vi "ArdnoFeed.vi"(0 "LINX Resource":T2={"IO"=enum."Remote", "Interface"=enum."Serial", "LINX Device Config"={"Interface"=enum."Serial", "COM Port"="COM13", "TCP Configuration"={"IP Address"="", "Port"=0}, "Device Family"=1, "Device ID"=1, "Device Name"="myRIO-1900", "TCP Ref"=refnum, "Channels"={"DI"=[0, 1, 2, 3, 4, 5, 6, 7, 8, 9, 10, 11, 12, 13, 14, 15, 16, 17, 18, 19, 20, 21, 22, 23, 24, 25, 26, 27, 28, 29, 30, 31, 32, 33, 34, 35, 36, 37, 38, 39, 40, 41, 42, 43, 44, 45, 46], "DO"=[0, 1, 2, 3, 4, 5, 6, 7, 8, 9, 10, 11, 12, 13, 14, 15, 16, 17, 18, 19, 20, 21, 22, 23, 24, 25, 26, 27, 28, 29, 30, 31, 32, 33, 34, 35, 36, 37, 38, 39, 40, 41, 42, 43, 44, 45, 46], "AI"=[0, 1, 2, 3, 4, 5, 6, 7, 8, 9, 10, 11], "AO"=[], "PWM"=[3, 5, 6, 9, 10], "QE"=[], "UART"=[0, 1], "I2C 2"=[0], "SPI"=[0], "CAN"=[], "Servo"=[], "AI Ref (V)"=0.0, "AI Resolution (Bits)"=0, "AO Ref (V)"=0.0, "AO Resolution (Bits)"=0}}}, 1 "chip selector":u16(ring) items=["8-Ring", "OneRing", "valveGR"], 5 "Reagent":u32, 7 "Ring":u16, 9 "Feed Cycles":i32, 11 "error in (no error)":errorcluster, 12 "All Rings":bool) -> (4 "LINX Resource out":T2, 6 "Elapsed [ms]":u32, 14 "ValveStates":bool[](array[boolean]), 15 "error out":errorcluster)   [LabVIEW 2018, in "Arduino.lvlib"]
uses:
  Arduino.lvlib
  <vilib>/MakerHub/LINX/Private/Type Defs/LINX Ref.ctl
  <vilib>/MakerHub/LINX/Private/Type Defs/Platform.ctl
  <vilib>/MakerHub/LINX/Private/Type Defs/Interface.ctl
  <vilib>/MakerHub/LINX/Private/Device/Type Defs/LINX Device Config.ctl
  <vilib>/MakerHub/LINX/Private/Device/Type Defs/TCP Config.ctl
  <vilib>/MakerHub/LINX/Private/Device/Type Defs/Channels.ctl
  <vilib>/MakerHub/LINX/Public/Peripherals/Digital/Digital Write N Chans.vi
  <vilib>/MakerHub/LINX/Private/Local IO/LinxDigitalWrite.vi
  <vilib>/MakerHub/LINX/Public/Utilities/Check Channel.vi
  <vilib>/MakerHub/LINX/Private/Utilties/Generate Error.vi
  <vilib>/MakerHub/LINX/LMH-LINX.lvlib
  <vilib>/MakerHub/LINX/Private/Device/Device.lvlib
panel:
  in  "ValveManualCluster":T1
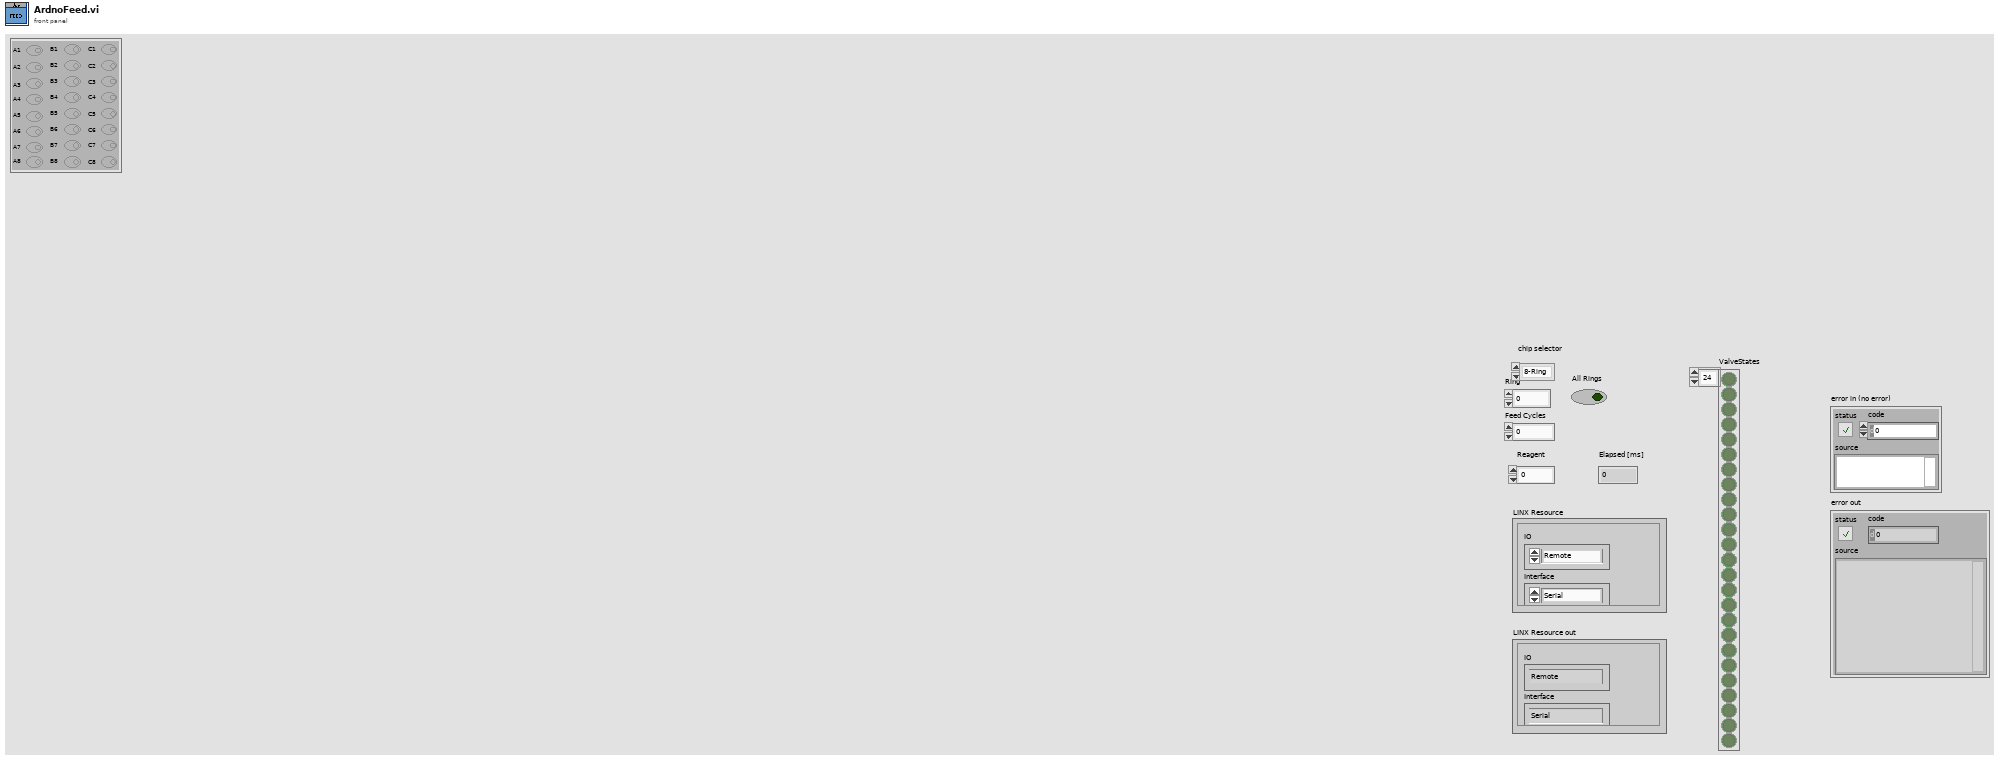
[diagram p1: front panel]
types:
  T1 = cluster{"C8":bool, "C7":bool, "C6":bool, "C5":bool, "C4":bool, "C3":bool, "C2":bool, "C1":bool, "B8":bool, "B7":bool, "B6":bool, "B5":bool, "B4":bool, "B3":bool, "B2":bool, "B1":bool, "A8":bool, "A7":bool, "A6":bool, "A5":bool, "A4":bool, "A3":bool, "A2":bool, "A1":bool}
  T2 = typedef "LMH-LINX.lvlib/LINX Ref.ctl" = cluster{"IO":T3, "Interface":T4, "LINX Device Config":T5}
  T3 = typedef "LMH-LINX.lvlib/Platform.ctl" = enum16{"Remote", "Local"}
  T4 = typedef "LMH-LINX.lvlib/Interface.ctl" = enum16{"Serial", "TCP"}
  T5 = typedef "LMH-LINX.lvlib/Device.lvlib/LINX Device Config.ctl" = cluster{"Interface":T4, "COM Port":refnum<visa-resource-name>, "TCP Configuration":T6, "Device Family":u8, "Device ID":u8, "Device Name":string, "TCP Ref":refnum<k5>, "Channels":T7}
  T6 = typedef "LMH-LINX.lvlib/Device.lvlib/TCP Config.ctl" = cluster{"IP Address":string, "Port":u16}
  T7 = typedef "LMH-LINX.lvlib/Channels.ctl" = cluster{"DI":u8[], "DO":u8[], "AI":u8[], "AO":u8[], "PWM":u8[], "QE":u8[], "UART":u8[], "I2C 2":u8[], "SPI":u8[], "CAN":u8[], "Servo":u8[], "AI Ref (V)":dbl, "AI Resolution (Bits)":u8, "AO Ref (V)":dbl, "AO Resolution (Bits)":u8}
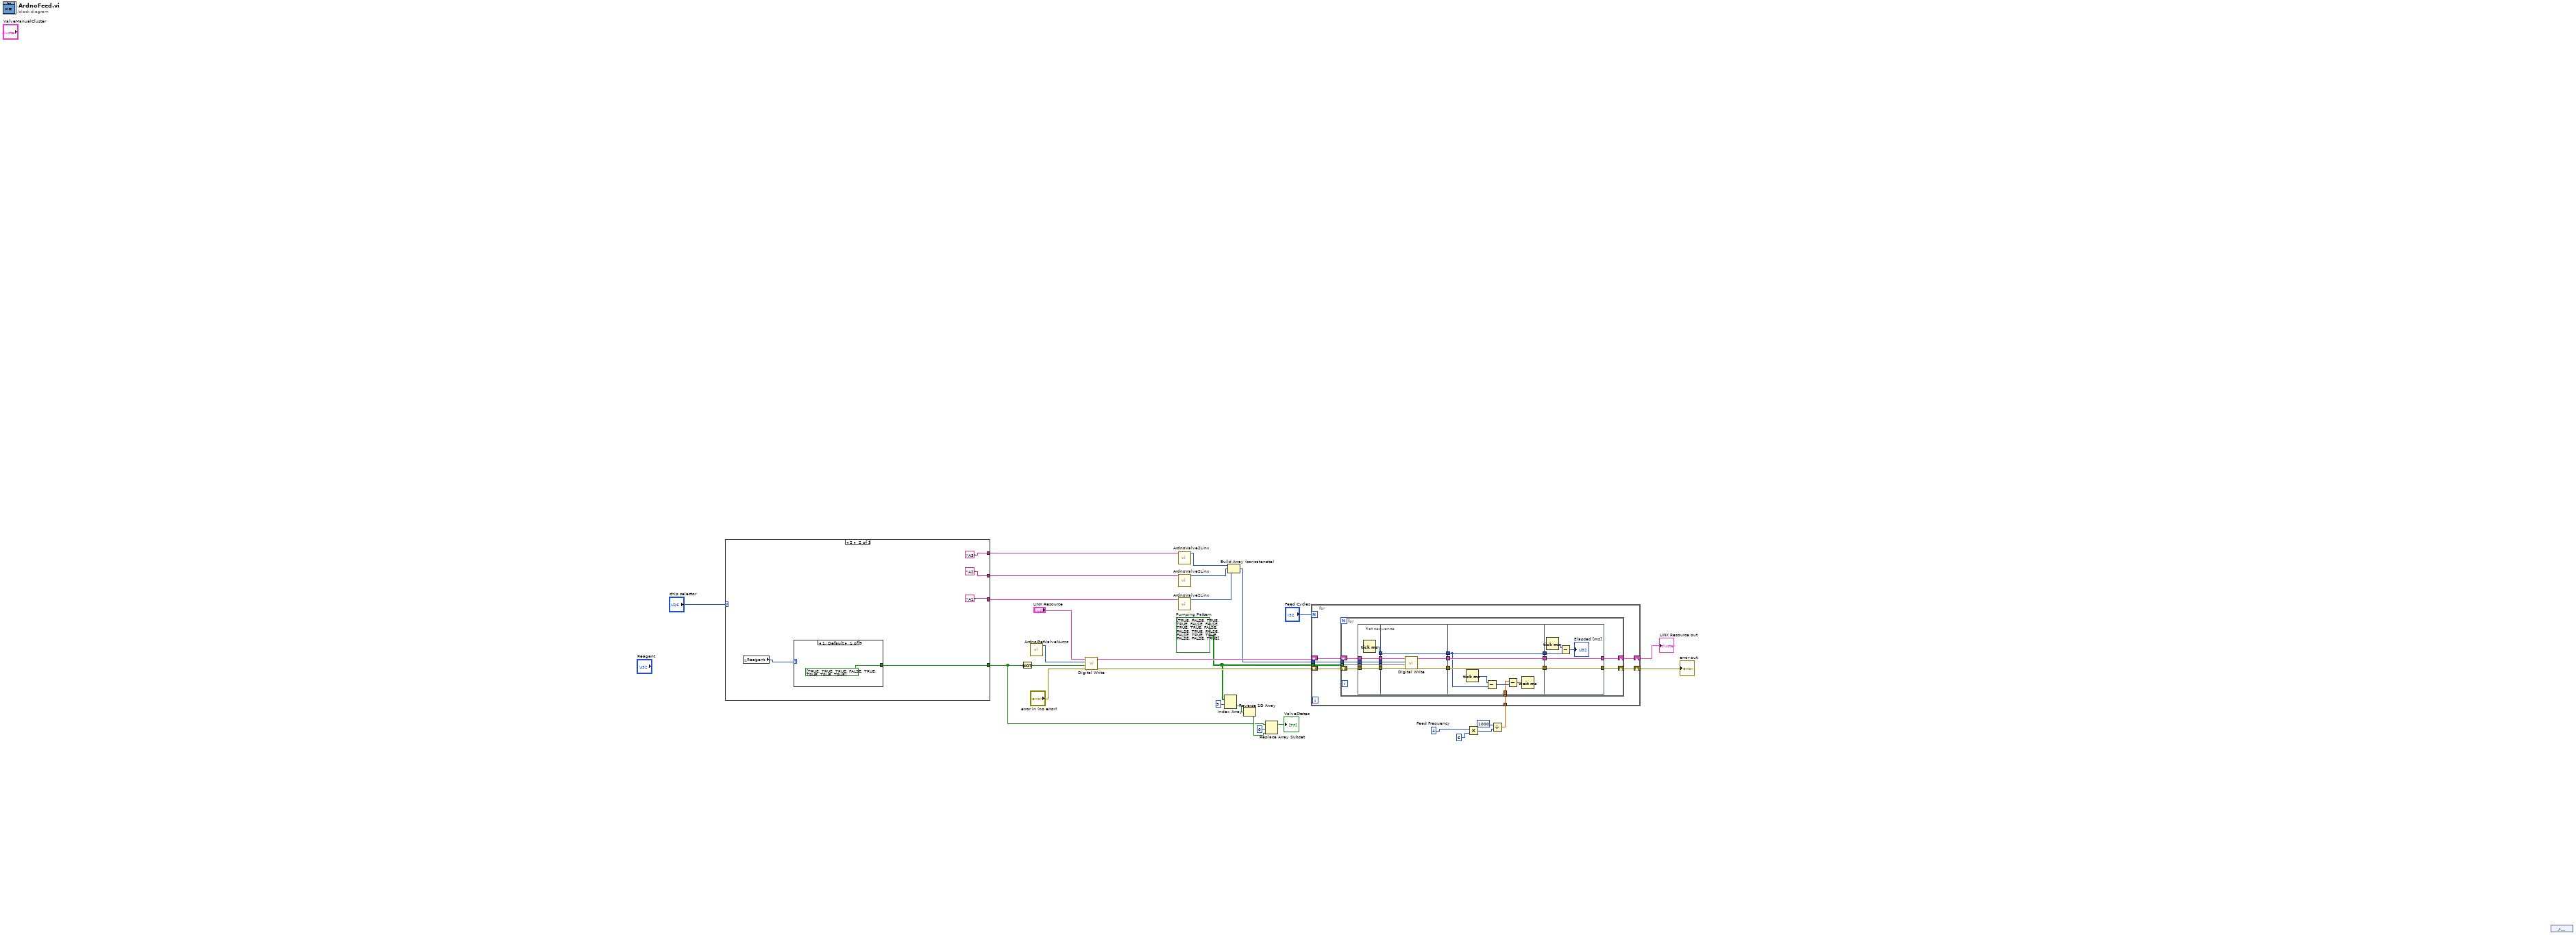
[diagram p0: block diagram]
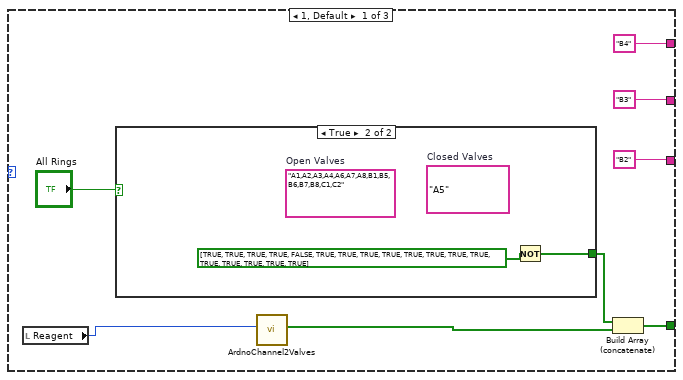
[diagram p2: hidden frame]
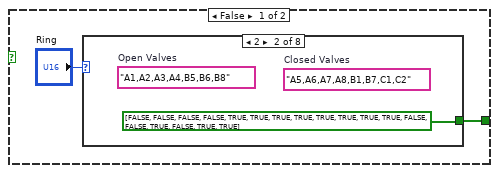
[diagram p3: hidden frame]
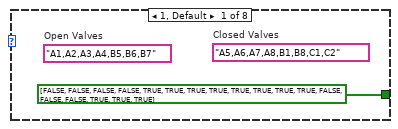
[diagram p4: hidden frame]
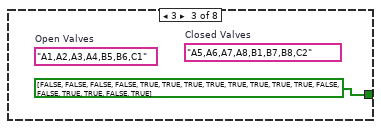
[diagram p5: hidden frame]
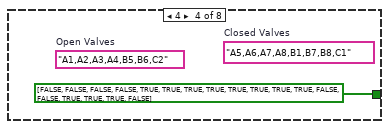
[diagram p6: hidden frame]
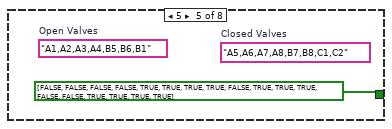
[diagram p7: hidden frame]
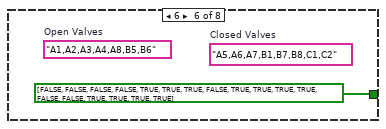
[diagram p8: hidden frame]
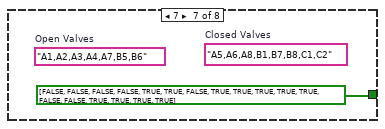
[diagram p9: hidden frame]
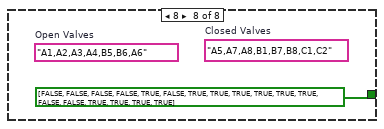
[diagram p10: hidden frame]
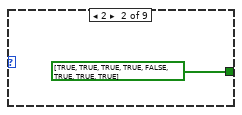
[diagram p11: hidden frame]
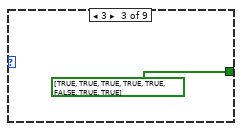
[diagram p12: hidden frame]
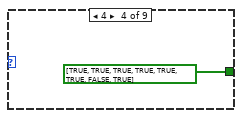
[diagram p13: hidden frame]
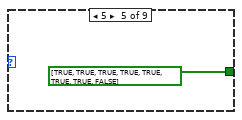
[diagram p14: hidden frame]
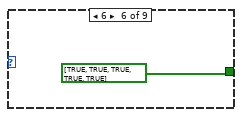
[diagram p15: hidden frame]
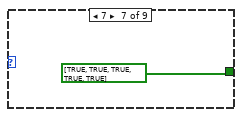
[diagram p16: hidden frame]
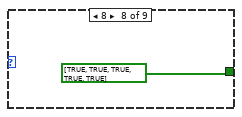
[diagram p17: hidden frame]
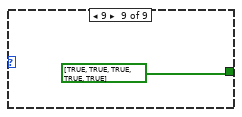
[diagram p18: hidden frame]
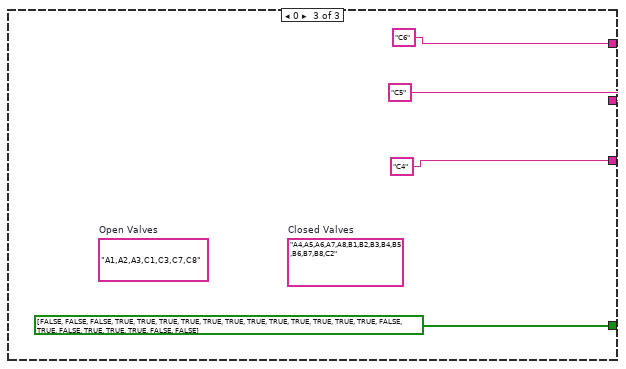
[diagram p19: hidden frame]
diagram:
  w19 = u32 4  # Feed Frequency
  w5 = bool[][] [[TRUE, FALSE, TRUE], [TRUE, FALSE, FALSE], [TRUE, TRUE, FALSE], [FALSE, TRUE, FALSE], [FALSE, TRUE, TRUE], [FALSE, FALSE, TRUE]]  # Pumping Pattern
  n1 = case shown="2" "chip selector" {
    tunnel: [w32 w50 bool[] [FALSE, FALSE, FALSE, TRUE, TRUE, TRUE, TRUE, TRUE, TRUE, TRUE, TRUE, TRUE, TRUE, TRUE, TRUE, FALSE, TRUE, FALSE, TRUE, TRUE, TRUE, FALSE, FALSE]] -> w4
    tunnel: ["B2" "A1" "C4"] -> w12
    tunnel: ["B3" "A2" "C5"] -> w11
    tunnel: ["B4" "A3" "C6"] -> w10
    frame 1, Default {
      n2 = local read "Reagent"() -> (w30:u32)
      n3 = case shown="True" "All Rings" {
        tunnel: [w38 w48] -> w36
        frame False {
          n4 = case shown="2" "Ring" {
            tunnel: [bool[] [FALSE, FALSE, FALSE, FALSE, TRUE, TRUE, TRUE, TRUE, TRUE, TRUE, TRUE, TRUE, FALSE, FALSE, FALSE, TRUE, TRUE, TRUE] bool[] [FALSE, FALSE, FALSE, FALSE, TRUE, TRUE, TRUE, TRUE, TRUE, TRUE, TRUE, TRUE, FALSE, FALSE, TRUE, FALSE, TRUE, TRUE] bool[] [FALSE, FALSE, FALSE, FALSE, TRUE, TRUE, TRUE, TRUE, TRUE, TRUE, TRUE, TRUE, FALSE, FALSE, TRUE, TRUE, FALSE, TRUE] bool[] [FALSE, FALSE, FALSE, FALSE, TRUE, TRUE, TRUE, TRUE, TRUE, TRUE, TRUE, TRUE, FALSE, FALSE, TRUE, TRUE, TRUE, FALSE] bool[] [FALSE, FALSE, FALSE, FALSE, TRUE, TRUE, TRUE, TRUE, FALSE, TRUE, TRUE, TRUE, FALSE, FALSE, TRUE, TRUE, TRUE, TRUE] bool[] [FALSE, FALSE, FALSE, FALSE, TRUE, TRUE, TRUE, FALSE, TRUE, TRUE, TRUE, TRUE, FALSE, FALSE, TRUE, TRUE, TRUE, TRUE] bool[] [FALSE, FALSE, FALSE, FALSE, TRUE, TRUE, FALSE, TRUE, TRUE, TRUE, TRUE, TRUE, FALSE, FALSE, TRUE, TRUE, TRUE, TRUE] bool[] [FALSE, FALSE, FALSE, FALSE, TRUE, FALSE, TRUE, TRUE, TRUE, TRUE, TRUE, TRUE, FALSE, FALSE, TRUE, TRUE, TRUE, TRUE]] -> w38
            frame 1, Default {
              (unwired) "A5,A6,A7,A8,B1,B8,C1,C2"  # Closed Valves
              (unwired) "A1,A2,A3,A4,B5,B6,B7"  # Open Valves
            }
            frame 2 {
              (unwired) "A5,A6,A7,A8,B1,B7,C1,C2"  # Closed Valves
              (unwired) "A1,A2,A3,A4,B5,B6,B8"  # Open Valves
            }
            frame 3 {
              (unwired) "A5,A6,A7,A8,B1,B7,B8,C2"  # Closed Valves
              (unwired) "A1,A2,A3,A4,B5,B6,C1"  # Open Valves
            }
            frame 4 {
              (unwired) "A5,A6,A7,A8,B1,B7,B8,C1"  # Closed Valves
              (unwired) "A1,A2,A3,A4,B5,B6,C2"  # Open Valves
            }
            frame 5 {
              (unwired) "A5,A6,A7,A8,B7,B8,C1,C2"  # Closed Valves
              (unwired) "A1,A2,A3,A4,B5,B6,B1"  # Open Valves
            }
            frame 6 {
              (unwired) "A5,A6,A7,B1,B7,B8,C1,C2"  # Closed Valves
              (unwired) "A1,A2,A3,A4,A8,B5,B6"  # Open Valves
            }
            frame 7 {
              (unwired) "A5,A6,A8,B1,B7,B8,C1,C2"  # Closed Valves
              (unwired) "A1,A2,A3,A4,A7,B5,B6"  # Open Valves
            }
            frame 8 {
              (unwired) "A5,A7,A8,B1,B7,B8,C1,C2"  # Closed Valves
              (unwired) "A1,A2,A3,A4,B5,B6,A6"  # Open Valves
            }
          }
        }
        frame True {
          (unwired) "A5"  # Closed Valves
          (unwired) "A1,A2,A3,A4,A6,A7,A8,B1,B5,B6,B7,B8,C1,C2"  # Open Valves
          n5 = Not(x=bool[] [TRUE, TRUE, TRUE, TRUE, FALSE, TRUE, TRUE, TRUE, TRUE, TRUE, TRUE, TRUE, TRUE, TRUE, TRUE, TRUE, TRUE, TRUE]) -> (.not. x?=w48:bool[])
        }
      }
      n6 = call "ArdnoChannel2Valves.vi"("Reagent"=w30) -> ("Valve State"=w31:bool[])  [unwired: 9 in]
      n7 = Build Array (concatenate)(w36, w31) -> (w32:bool[])
    }
    frame 2 {
      n8 = local read "Reagent"() -> (w51:u32)
      n9 = case shown="1, Default" w51 {
        tunnel: [bool[] [TRUE, TRUE, TRUE, FALSE, TRUE, TRUE, TRUE, TRUE] bool[] [TRUE, TRUE, TRUE, TRUE, FALSE, TRUE, TRUE, TRUE] bool[] [TRUE, TRUE, TRUE, TRUE, TRUE, FALSE, TRUE, TRUE] bool[] [TRUE, TRUE, TRUE, TRUE, TRUE, TRUE, FALSE, TRUE] bool[] [TRUE, TRUE, TRUE, TRUE, TRUE, TRUE, TRUE, FALSE] bool[] [TRUE, TRUE, TRUE, TRUE, TRUE] bool[] [TRUE, TRUE, TRUE, TRUE, TRUE] bool[] [TRUE, TRUE, TRUE, TRUE, TRUE] bool[] [TRUE, TRUE, TRUE, TRUE, TRUE]] -> w50
        frame 1, Default {
        }
        frame 2 {
        }
        frame 3 {
        }
        frame 4 {
        }
        frame 5 {
        }
        frame 6 {
        }
        frame 7 {
        }
        frame 8 {
        }
        frame 9 {
        }
      }
    }
    frame 0 {
      (unwired) "A4,A5,A6,A7,A8,B1,B2,B3,B4,B5,B6,B7,B8,C2"  # Closed Valves
      (unwired) "A1,A2,A3,C1,C3,C7,C8"  # Open Valves
    }
  }
  n10 = Not(x=w4) -> (.not. x?=w1:bool[])
  n11 = call "ArdnoGetValveNums.vi"() -> ("Array"=w2:i32[])  [unwired: 11 in]
  n12 = call-poly <vilib>:"Digital Write.vi"("Error In"="error in (no error)", "Values"=w1, "DO Channels"=w2, "LINX Resource"="LINX Resource") -> ("Error Out"=w24:errorcluster, "LINX Resource"=w23:T2)  [unwired: 6 in]
  n13 = call "ArdnoValve2Linx.vi"("Valve (A1-C8),\n comma separated"=w10) -> ("Linx Port"=w13:i32[])  [unwired: 8 in, 2 out]
  n14 = call "ArdnoValve2Linx.vi"("Valve (A1-C8),\n comma separated"=w11) -> ("Linx Port"=w14:i32[])  [unwired: 8 in, 2 out]
  n15 = call "ArdnoValve2Linx.vi"("Valve (A1-C8),\n comma separated"=w12) -> ("Linx Port"=w15:i32[])  [unwired: 8 in, 2 out]
  n16 = Index Array(array=w5, index (row)=5) -> (element=w8:bool[])  [unwired: 1 in]
  n17 = Build Array (concatenate)(w13, w14, w15) -> (w18:i32[])
  n18 = Reverse 1D Array(array=w8) -> (reversed array=w7:bool[])
  n19 = Replace Array Subset(array=w4, new element=w7, index=0) -> (→"ValveStates":bool[])
  n20 = Multiply(x=w19, y=u32 6) -> (x*y=w25:u32)
  n21 = Divide(x=u32 1000, y=w25) -> (x/y=w26:dbl)
  n22 = for {
    N: "Feed Cycles" -> [_]
    tunnel: w18 -> [w72]
    tunnel: w5 -> [w71]
    shift-right: [w70] -> w22
    shift-left: w23 -> [w74]
    shift-right: [w69] -> w21
    shift-left: w24 -> [w73]
    tunnel: w26 -> [w68]
    n23 = for {
      tunnel: w71 -> [w87] mode=indexing
      tunnel: w72 -> [w90]
      shift-right: [w89] -> w70
      shift-left: w74 -> [w92]
      shift-right: [w88] -> w69
      shift-left: w73 -> [w91]
      tunnel: w68 -> [w78]
      n24 = flat-sequence {
        tunnel: w87 -> [w94]
        tunnel: w90 -> [w95]
        tunnel: w91 -> [w96]
        tunnel: w92 -> [w97]
        tunnel: [w97] -> w86
        tunnel: [w96] -> w85
        tunnel: [w95] -> w84
        tunnel: [w94] -> w83
        tunnel: [w93] -> w82
        tunnel: [w101] -> w77
        tunnel: [w100] -> w76
        tunnel: w86 -> [w104]
        tunnel: w85 -> [w103]
        tunnel: w84 -> [w102]
        tunnel: w83 -> [w99]
        tunnel: w82 -> [w98]
        tunnel: [w98] -> w75
        tunnel: w77 -> [w111]
        tunnel: w76 -> [w110]
        tunnel: w75 -> [w108]
        tunnel: [w111] -> w81
        tunnel: [w110] -> w80
        tunnel: [w108] -> w79
        tunnel: w78 -> [w105]
        tunnel: [w115] -> w88
        tunnel: [w116] -> w89
        tunnel: w81 -> [w116]
        tunnel: w80 -> [w115]
        tunnel: w79 -> [w112]
        frame #0 {
          n25 = Tick Count (ms)() -> (millisecond timer value=w93:u32)
        }
        frame #1 {
          n26 = call-poly <vilib>:"Digital Write.vi"("Error In"=w103, "Values"=w99, "DO Channels"=w102, "LINX Resource"=w104) -> ("Error Out"=w100:errorcluster, "LINX Resource"=w101:T2)  [unwired: 6 in]
        }
        frame #2 {
          n27 = Tick Count (ms)() -> (millisecond timer value=w109:u32)
          n28 = Subtract(x=w109, y=w108) -> (x-y=w107:u32)
          n29 = Subtract(x=w105, y=w107) -> (x-y=w106:dbl)
          n30 = Wait (ms)(milliseconds to wait=w106) -> ()  [unwired: 1 out]
        }
        frame #3 {
          n31 = Tick Count (ms)() -> (millisecond timer value=w113:u32)
          n32 = Subtract(x=w113, y=w112) -> (x-y=→"Elapsed [ms]":u32)
        }
      }
    }
  }
  "error out" <- w21
  "LINX Resource out" <- w22
  n33 = control-ref of="ValveManualCluster"() -> ()  [unwired: 1 out]
